vi "Example_BulkCapture.vi"() -> ()   [LabVIEW 2021, in "BrainStem2_LabVIEW_Library.lvlib"]
uses:
  BrainStem2_LabVIEW_Library.lvlib
panel:
  out "16 Bit Combined Data":u16[](array[numeric])
  out "Raw Slot Output (8 Bit Values)":u8[](array[numeric])
  out "Number of Bytes Unloaded":dbl
  out "Number of Bytes TO Unload":dbl
  out "Bulk Capture Status":string
  in  "Sample Rate":u32=7000 min=7000 max=200000
  in  "Number of Samples":u32=1 min=1 max=8000
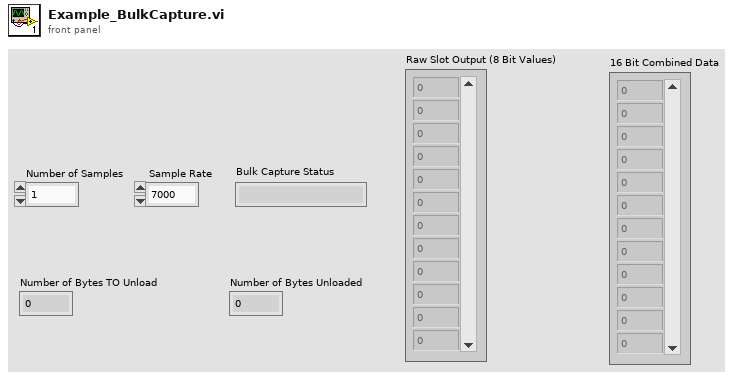
[diagram p1: front panel]
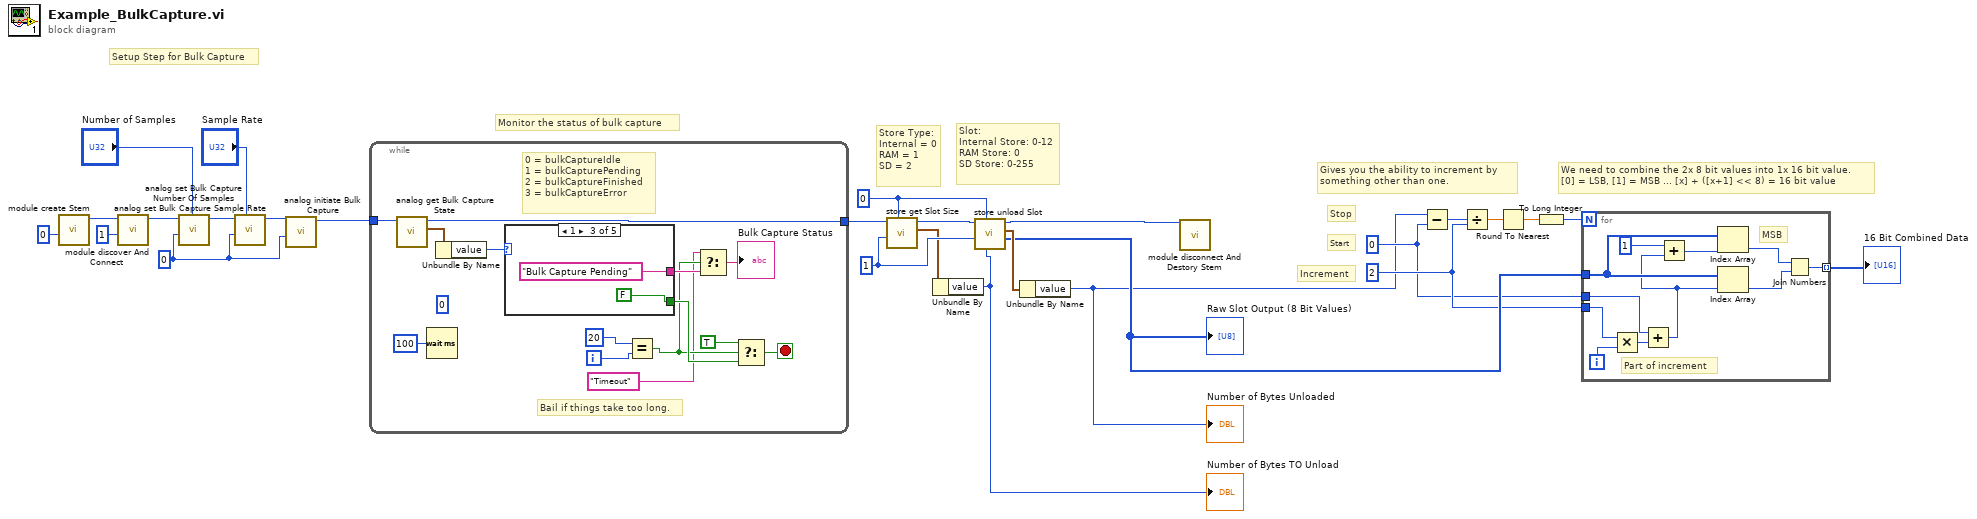
[diagram p0: block diagram]
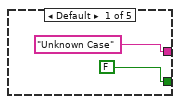
[diagram p2: hidden frame]
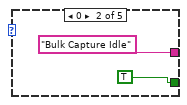
[diagram p3: hidden frame]
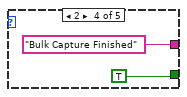
[diagram p4: hidden frame]
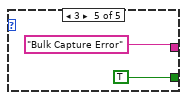
[diagram p5: hidden frame]
diagram:
  w4 = 2 ("x")
  w3 = 0 ("x")
  w15 = 1 ("storeType")
  w16 = 0 ("slot")
  w18 = 0 ("analogNum")
  # "Monitor the status of bulk capture"
  # "Setup Step for Bulk Capture"
  # "We need to combine the 2x 8 bit values into 1x 16 bit value.\n[0] = LSB, [1] = MSB ... [x] + ([x+1] << 8) = 16 bit value"
  # "Gives you the ability to increment by \nsomething other than one."
  # "Stop"
  # "Increment"
  # "Start"
  # "Slot:\nInternal Store: 0-12\nRAM Store: 0\nSD Store: 0-255"
  # "Store Type:\nInternal = 0\nRAM = 1\nSD = 2"
  n1 = call "module create Stem.vi"("sn"=u32 0) -> ("id out"=w27:u32)  [unwired: 8 in, 2 out]
  n2 = call "module discover And Connect.vi"("transport"=1, "id"=w27) -> ("id out"=w24:u32)  [unwired: 7 in, 2 out]
  n3 = call "analog set Bulk Capture Number Of Samples.vi"("value"="Number of Samples", "index"=w18, "id"=w24) -> ("id out"=w22:u32)  [unwired: 6 in, 2 out]
  n4 = call "analog set Bulk Capture Sample Rate.vi"("value"="Sample Rate", "index"=w18, "id"=w22) -> ("id out"=w20:u32)  [unwired: 6 in, 2 out]
  n5 = call "analog initiate Bulk Capture.vi"("index"=w18, "id"=w20) -> ("id out"=w19:u32)  [unwired: 7 in, 2 out]
  n6 = while {
    tunnel: w19 -> [w34]
    tunnel: [w33] -> w17
    i -> [w39]
    stop <- w35 stop-if-true
    (unwired) 0
    # "Bail if things take too long."
    # "0 = bulkCaptureIdle\n1 = bulkCapturePending\n2 = bulkCaptureFinished\n3 = bulkCaptureError"
    n7 = call "analog get Bulk Capture State.vi"("id"=w34) -> ("result out"=w41:cluster{"value":i32, "error":i32}, "id out"=w33:u32)  [unwired: 8 in, 1 out]
    n8 = Wait (ms)(milliseconds to wait=u32 100) -> ()  [unwired: 1 out]
    n9 = Unbundle By Name(w41) -> ("value"=w32:i32)
    n10 = case shown="1" w32 {
      tunnel: ["Unknown Case" "Bulk Capture Idle" "Bulk Capture Pending" "Bulk Capture Finished" "Bulk Capture Error"] -> w31
      tunnel: [FALSE TRUE FALSE TRUE TRUE] -> w37
      frame Default {
      }
      frame 0 {
      }
      frame 1 {
      }
      frame 2 {
      }
      frame 3 {
      }
    }
    n11 = Equal?(x=20, y=w39) -> (x = y?=w30:bool)
    n12 = Select(t="Timeout", s=w30, f=w31) -> (s? t:f=→"Bulk Capture Status":string)
    n13 = Select(t=TRUE, s=w30, f=w37) -> (s? t:f=w35:bool)
  }
  n14 = call "store get Slot Size.vi"("slot"=w16, "index"=w15, "id"=w17) -> ("result out"=w13:cluster{"value":i32, "error":i32}, "id out"=w14:u32)  [unwired: 6 in, 1 out]
  n15 = Unbundle By Name(w13) -> ("value"=w12:i32)
  "Number of Bytes TO Unload" <- w12
  n16 = call "store unload Slot.vi"("bufferLength"=w12, "slot"=w16, "index"=w15, "id"=w14) -> ("buffer"=w5:u8[], "result out"=w11:cluster{"value":i32, "error":i32}, "id out"=w10:u32)  [unwired: 4 in, 1 out]
  "Raw Slot Output (8 Bit Values)" <- w5
  n17 = Unbundle By Name(w11) -> ("value"=w1:i32)
  "Number of Bytes Unloaded" <- w1
  n18 = call "module disconnect And Destory Stem.vi"("id"=w10) -> ()  [unwired: 8 in, 3 out]
  n19 = Subtract(x=w1, y=w3) -> (x-y=w9:i32)
  n20 = Divide(x=w9, y=w4) -> (x/y=w8:dbl)
  n21 = Round To Nearest(number=w8) -> (nearest integer value=w7:dbl)
  n22 = To Long Integer(number=w7) -> (32bit integer=w6:i32)
  n23 = for {
    N: w6 -> [_]
    tunnel: w4 -> [w61]
    tunnel: w3 -> [w59]
    tunnel: w5 -> [w57]
    tunnel: [w56] -> w2 mode=indexing
    i -> [w62]
    # "MSB"
    # "Part of increment"
    n24 = Multiply(x=w61, y=w62) -> (x*y=w60:i32)
    n25 = Add(x=w59, y=w60) -> (x+y=w52:i32)
    n26 = Add(x=1 ("y"), y=w52) -> (x+y=w58:i32)
    n27 = Index Array(array=w57, index=w58) -> (element=w55:u8)
    n28 = Index Array(array=w57, index=w52) -> (element=w54:u8)
    n29 = Join Numbers(hi=w55, lo=w54) -> ((hi.lo)=w56:u16)
  }
  "16 Bit Combined Data" <- w2
